vi "config_TRIG.vi"(10 "VISA resource name":refnum<visa-resource-name>="TRIG") -> (0 "duration ind.":dbl[](array[numeric]) min=0.0 format="%.3f", 1 "start time ind.":dbl[](array[numeric]) format="%.3f", 2 "delay data in TRIG":dbl[](array[numeric]) caption="delay array" min=0.0 max=2000.0 format="%05.2p")   [LabVIEW 2011]
uses:
  <vilib>/Platform/browser.llb/Open URL in Default Browser (string).vi
  global.vi
panel:
  out "fast wave":bool
  in  "burst period":dbl
  in  "burst count":i32
  in  "help":bool
  in  "AWG":bool
  in  "SWITCH":bool
  in  "OSC":bool
  in  "Power Amp":bool
  in  "Nozzle":bool
  in  "duration":dbl[](array[numeric]) min=0.0 format="%.3f"
  in  "start time":dbl[](array[numeric]) format="%.3f"
  in  "time unit":enum16{"s", "ms", "us", "ns"}(ring)=enum."us"
  in  "write config":bool
  in  "read delay data":bool
  in  "display resolution":i32=100
  out "Digital Waveform Graph":digitalwaveform(graph)
  in  "stop":bool
  # "Configure Delay Generator"
  # "Polarity"
  # "NEGATIVE"
  # "POSITIVE"
  # "Nozzle"
  # "power AMP"
  # "AWG"
  # "SWITCH"
  # "OSC"
  # "t0"
  # "t"
  # "A"
  # "B"
  # "C"
  # "D"
  # "E"
  # "F"
  # "G"
  # "H"
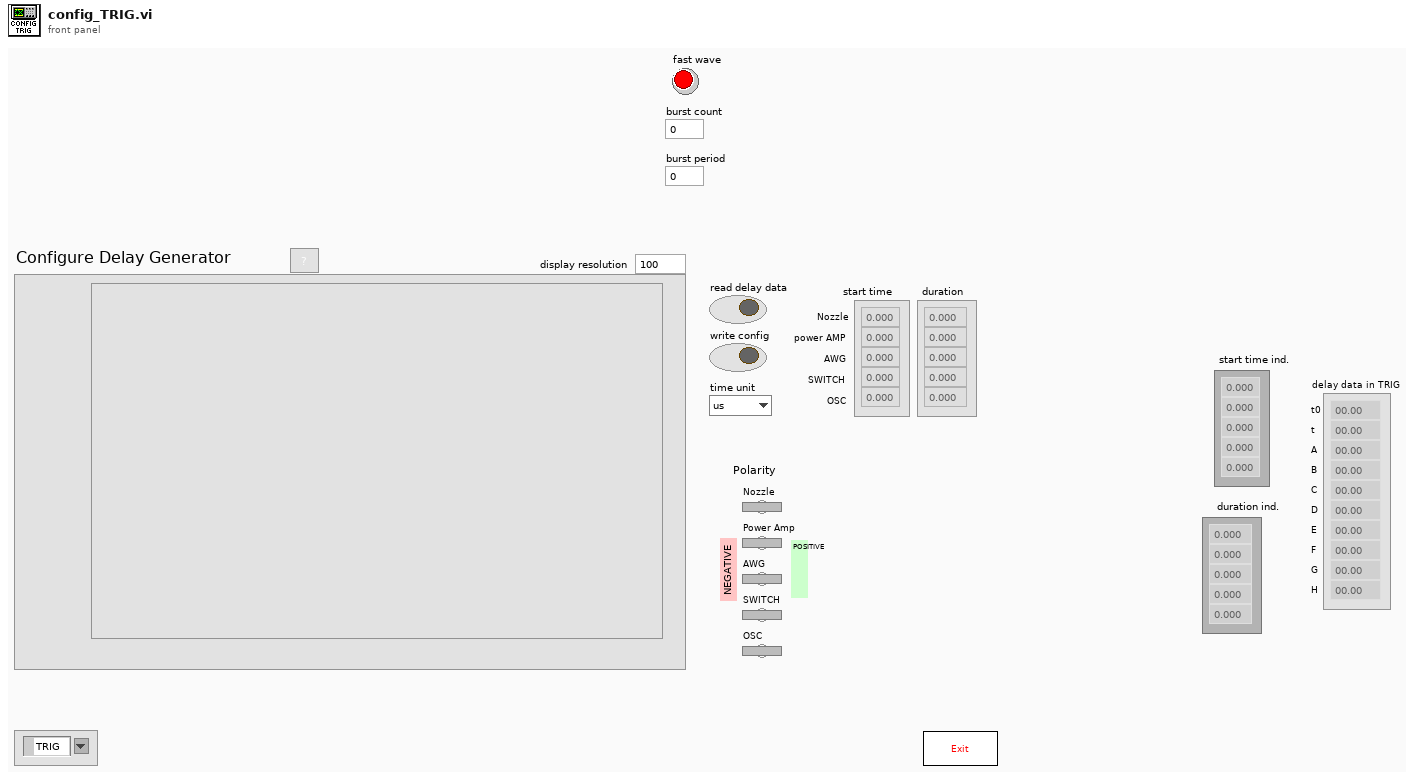
[diagram p1: front panel]
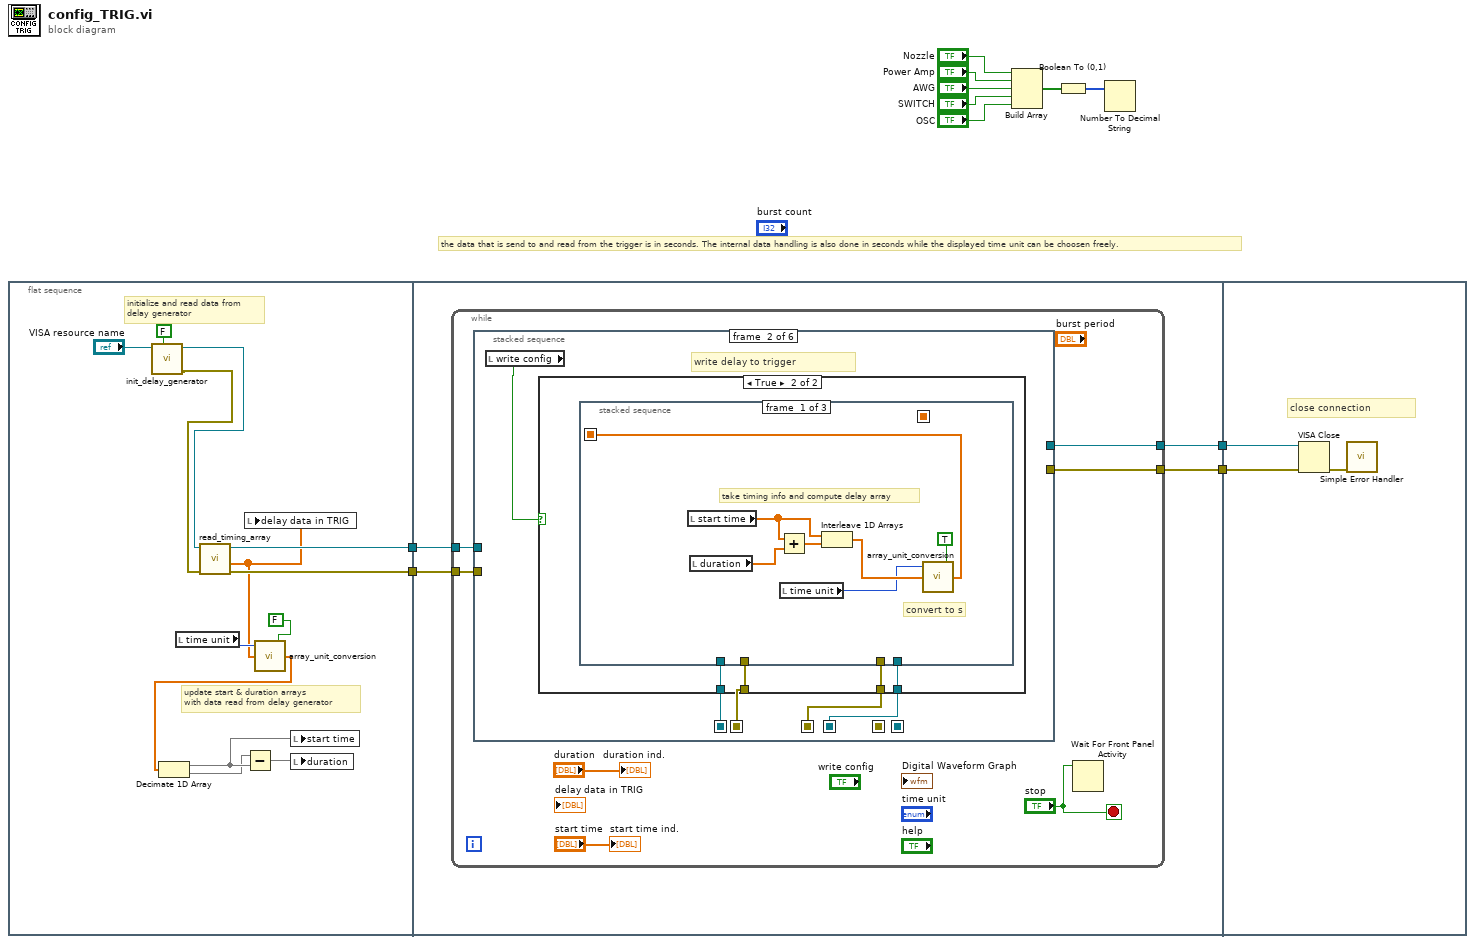
[diagram p0: block diagram]
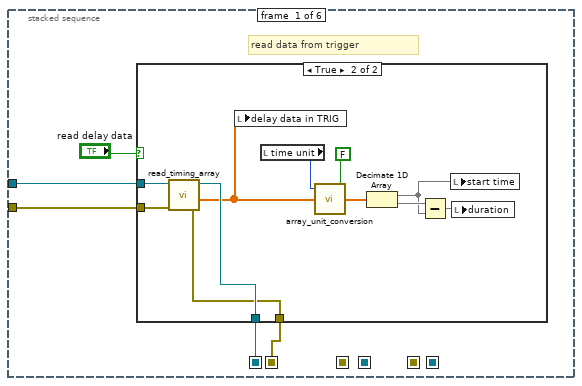
[diagram p2: hidden frame]
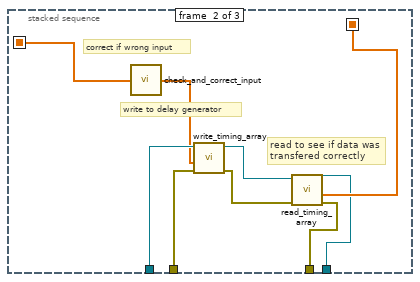
[diagram p5: hidden frame]
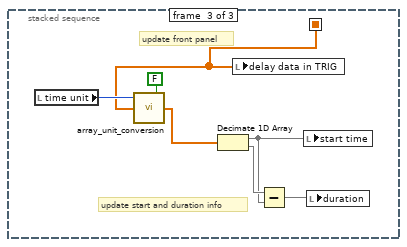
[diagram p6: hidden frame]
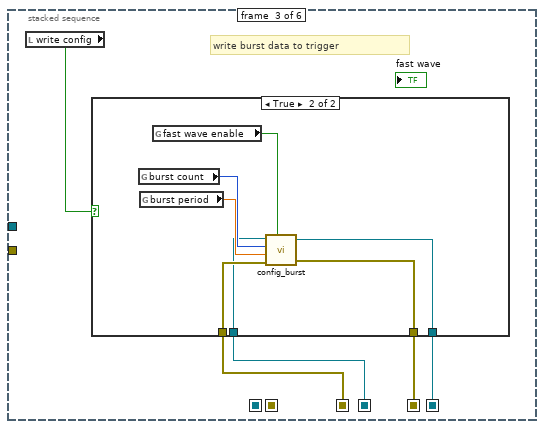
[diagram p7: hidden frame]
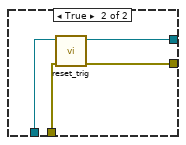
[diagram p10: hidden frame]
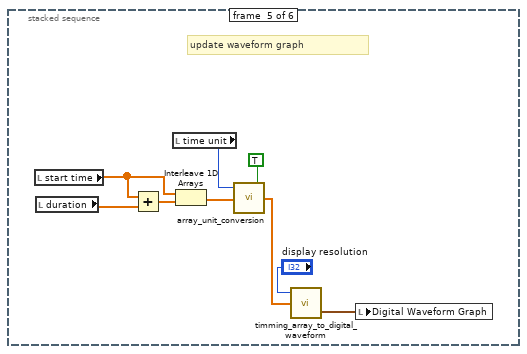
[diagram p11: hidden frame]
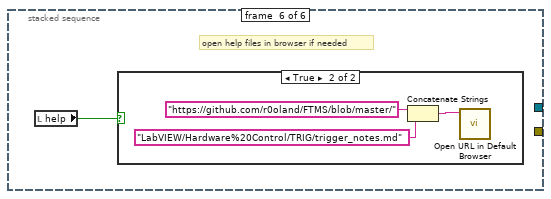
[diagram p12: hidden frame]
diagram:
  # "the data that is send to and read from the trigger is in seconds. The internal data handling is also done in seconds while the displayed time unit can be choosen freely."
  n1 = flat-sequence {
    tunnel: [w23] -> w11
    tunnel: [w24] -> w10
    tunnel: w11 -> [w28]
    tunnel: w10 -> [w27]
    tunnel: [w26] -> w9
    tunnel: [w25] -> w8
    tunnel: w9 -> [w127]
    tunnel: w8 -> [w126]
    frame #0 {
      # "update start & duration arrays \nwith data read from delay generator"
      # "initialize and read data from \ndelay generator"
      n2 = call "init_delay_generator.vi"("reset TRIG"=FALSE, "VISA resource name"="VISA resource name") -> ("error out"=w14:errorcluster, "VISA resource name out"=w15:refnum<visa-resource-name>)  [unwired: 5 in]
      n3 = local read "time unit"() -> (w20:enum16{"s", "ms", "us", "ns"})
      n4 = call "read_timing_array.vi"("error in"=w14, "VISA resource in"=w15) -> ("error out 2"=w24:errorcluster, "delay array"=w19:dbl[], "VISA resource out"=w23:refnum<visa-resource-name>)  [unwired: 3 in]
      n5 = local write "delay data in TRIG"(w19) -> ()
      n6 = call "array_unit_conversion.vi"("inverse function (arb. unit to s)?"=FALSE, "delay array"=w19, "time unit"=w20) -> ("output"=w18:dbl[])  [unwired: 2 in]
      n7 = Decimate 1D Array(w18) -> (w21:dbl[], w16:dbl[])
      n8 = Subtract(x=w16, y=w21) -> (x-y=w22:dbl[])
      n9 = local write "start time"(w21) -> ()
      n10 = local write "duration"(w22) -> ()
    }
    frame #1 {
      n11 = while {
        tunnel: w27 -> [w33]
        tunnel: [w35] -> w26
        tunnel: [w34] -> w25
        tunnel: w28 -> [w31]
        stop <- "stop" stop-if-true
        n12 = stacked-sequence {
          seq-local: [w38 _ _ _ _ _] -> [_ w58 _ _ _ _]
          seq-local: [w37 _ _ _ _ _] -> [_ w57 _ _ _ _]
          seq-local: [_ w56 _ _ _ _] -> [_ _ w91 _ _ _]
          seq-local: [_ w55 _ _ _ _] -> [_ _ w90 _ _ _]
          seq-local: [_ _ w88 _ _ _] -> [_ _ _ w105 _ _]
          seq-local: [_ _ w89 _ _ _] -> [_ _ _ w104 _ _]
          tunnel: w31 -> [w40 _ _ _ _ _]
          tunnel: w33 -> [w39 _ _ _ _ _]
          tunnel: [_ _ _ w102 _ _] -> w34
          tunnel: [_ _ _ w103 _ _] -> w35
          frame #0 {
            # "read data from trigger"
            n13 = case shown="True" "read delay data" {
              tunnel: w40 -> [w41 w53]
              tunnel: w39 -> [w42 w52]
              tunnel: [w41 w51] -> w38
              tunnel: [w42 w50] -> w37
              frame False {
              }
              frame True {
                n14 = call "read_timing_array.vi"("error in"=w52, "VISA resource in"=w53) -> ("error out 2"=w50:errorcluster, "delay array"=w43:dbl[], "VISA resource out"=w51:refnum<visa-resource-name>)  [unwired: 3 in]
                n15 = local write "delay data in TRIG"(w43) -> ()
                n16 = local read "time unit"() -> (w46:enum16{"s", "ms", "us", "ns"})
                n17 = call "array_unit_conversion.vi"("inverse function (arb. unit to s)?"=FALSE, "delay array"=w43, "time unit"=w46) -> ("output"=w44:dbl[])  [unwired: 2 in]
                n18 = Decimate 1D Array(w44) -> (w47:dbl[], w48:dbl[])
                n19 = Subtract(x=w48, y=w47) -> (x-y=w49:dbl[])
                n20 = local write "start time"(w47) -> ()
                n21 = local write "duration"(w49) -> ()
              }
            }
          }
          frame #1 {
            # "write delay to trigger"
            n22 = local read "write config"() -> (w54:bool)
            n23 = case shown="True" w54 {
              tunnel: w58 -> [w59 w64]
              tunnel: w57 -> [w60 w63]
              tunnel: [w60 w62] -> w56
              tunnel: [w59 w61] -> w55
              frame False {
              }
              frame True {
                n24 = stacked-sequence {
                  seq-local: [w65 _ _] -> [_ w76 _]
                  seq-local: [_ w74 _] -> [_ _ w83]
                  tunnel: w64 -> [_ w80 _]
                  tunnel: w63 -> [_ w79 _]
                  tunnel: [_ w73 _] -> w62
                  tunnel: [_ w72 _] -> w61
                  frame #0 {
                    # "convert to s"
                    # "take timing info and compute delay array"
                    n25 = local read "start time"() -> (w70:dbl[])
                    n26 = local read "duration"() -> (w69:dbl[])
                    n27 = Add(x=w70, y=w69) -> (x+y=w71:dbl[])
                    n28 = local read "time unit"() -> (w66:enum16{"s", "ms", "us", "ns"})
                    n29 = Interleave 1D Arrays(w70, w71) -> (w67:dbl[])
                    n30 = call "array_unit_conversion.vi"("inverse function (arb. unit to s)?"=TRUE, "delay array"=w67, "time unit"=w66) -> ("output"=w65:dbl[])  [unwired: 2 in]
                  }
                  frame #1 {
                    # "read to see if data was \ntransfered correctly"
                    # "write to delay generator"
                    # "correct if wrong input"
                    n31 = call "check_and_correct_input.vi"("delay array"=w76) -> ("corrrected delay array"=w75:dbl[])  [unwired: 4 in]
                    n32 = call "write_timing_array.vi"("error in"=w79, "delay array"=w75, "VISA resource in"=w80) -> ("error out 2"=w77:errorcluster, "VISA resource out"=w78:refnum<visa-resource-name>)  [unwired: 2 in, 1 out]
                    n33 = call "read_timing_array.vi"("error in"=w77, "VISA resource in"=w78) -> ("error out 2"=w73:errorcluster, "delay array"=w74:dbl[], "VISA resource out"=w72:refnum<visa-resource-name>)  [unwired: 3 in]
                  }
                  frame #2 {
                    # "update front panel"
                    # "update start and duration info"
                    n34 = local read "time unit"() -> (w84:enum16{"s", "ms", "us", "ns"})
                    n35 = call "array_unit_conversion.vi"("inverse function (arb. unit to s)?"=FALSE, "delay array"=w83, "time unit"=w84) -> ("output"=w82:dbl[])  [unwired: 2 in]
                    n36 = Decimate 1D Array(w82) -> (w85:dbl[], w87:dbl[])
                    n37 = local write "delay data in TRIG"(w83) -> ()
                    n38 = Subtract(x=w87, y=w85) -> (x-y=w86:dbl[])
                    n39 = local write "start time"(w85) -> ()
                    n40 = local write "duration"(w86) -> ()
                  }
                }
              }
            }
          }
          frame #2 {
            # "write burst data to trigger"
            n41 = local read "write config"() -> (w92:bool)
            n42 = case shown="True" w92 {
              tunnel: w91 -> [w93 w99]
              tunnel: w90 -> [w94 w98]
              tunnel: [w94 w97] -> w89
              tunnel: [w93 w96] -> w88
              frame False {
              }
              frame True {
                n43 = global read "global.vi" "burst count"() -> (w101:i32)
                n44 = global read "global.vi" "burst period"() -> (w100:dbl)
                n45 = global read "global.vi" "fast wave enable"() -> (w95:bool)
                n46 = call "config_burst.vi"("VISA resource name"=w98, "burst count"=w101, "burst period (s)"=w100, "error in (no error)"=w99, "Burst enable?"=w95) -> ("VISA resource name out"=w97:refnum<visa-resource-name>, "error out"=w96:errorcluster)  [unwired: 1 in]
              }
            }
          }
          frame #3 {
            # "rest instruments to default settings"
            n47 = case shown="False" {
              selector: _ -> [_ _]
              tunnel: w105 -> [w106 w111]
              tunnel: w104 -> [w107 w110]
              tunnel: [w107 w109] -> w103
              tunnel: [w106 w108] -> w102
              frame False {
              }
              frame True {
                n48 = call "reset_trig.vi"("error in (no error)"=w111, "VISA resource name"=w110) -> ("error out"=w108:errorcluster, "VISA resource name out"=w109:refnum<visa-resource-name>)  [unwired: 8 in]
              }
            }
          }
          frame #4 {
            # "update waveform graph"
            n49 = local read "start time"() -> (w114:dbl[])
            n50 = local read "duration"() -> (w113:dbl[])
            n51 = Add(x=w114, y=w113) -> (x+y=w118:dbl[])
            n52 = local read "time unit"() -> (w115:enum16{"s", "ms", "us", "ns"})
            n53 = Interleave 1D Arrays(w114, w118) -> (w116:dbl[])
            n54 = call "array_unit_conversion.vi"("inverse function (arb. unit to s)?"=TRUE, "delay array"=w116, "time unit"=w115) -> ("output"=w112:dbl[])  [unwired: 2 in]
            n55 = call "timming_array_to_digital_waveform.vi"("delay array"=w112, "resolution"="display resolution") -> ("digital waveform"=w120:digitalwaveform)  [unwired: 2 in]
            n56 = local write "Digital Waveform Graph"(w120) -> ()
          }
          frame #5 {
            # "open help files in browser if needed"
            n57 = local read "help"() -> (w121:bool)
            n58 = case shown="True" w121 {
              frame False {
              }
              frame True {
                n59 = Concatenate Strings("https://github.com/r0oland/FTMS/blob/master/" ("string"), "LabVIEW/Hardware%20Control/TRIG/trigger_notes.md" ("string")) -> (w124:string)
                n60 = call-poly <vilib>:"Open URL in Default Browser.vi"("URL"=w124) -> ()  [unwired: 5 in, 2 out]
              }
            }
          }
        }
        n61 = Wait For Front Panel Activity(3:"stop") -> ()  [unwired: 2 in, 1 out]
        "start time ind." <- "start time"
        "duration ind." <- "duration"
      }
    }
    frame #2 {
      # "close connection"
      n62 = VISA Close(VISA resource name=w127, error in (no error)=w126) -> (error out=w125:errorcluster)
      n63 = call <vilib>:"Simple Error Handler.vi"("error in (no error)"=w125) -> ()  [unwired: 4 in, 5 out]
    }
  }
  n64 = Build Array("Nozzle", "Power Amp", "AWG", "SWITCH", "OSC") -> (w7:bool[])
  n65 = Boolean To (0,1)(Boolean=w7) -> (0, 1=w6:i16[])
  n66 = Number To Decimal String(number=w6) -> ()  [unwired: 1 in, 1 out]
